vi "Read New Top Layer ID.vi"(8 "error in (no error)":errorcluster, 11 "Database Entry in":refnum<class "Database Entry.lvclass">) -> (0 "error out":errorcluster, 2 "Revised Sensor IDs":string[](array[string]), 3 "Database Entry out":refnum<class "Database Entry.lvclass">)   [LabVIEW 2021, in "Database Entry.lvclass"]
uses:
  Database Entry.lvclass
  Database Entry.lvclass/Database Entry.ctl
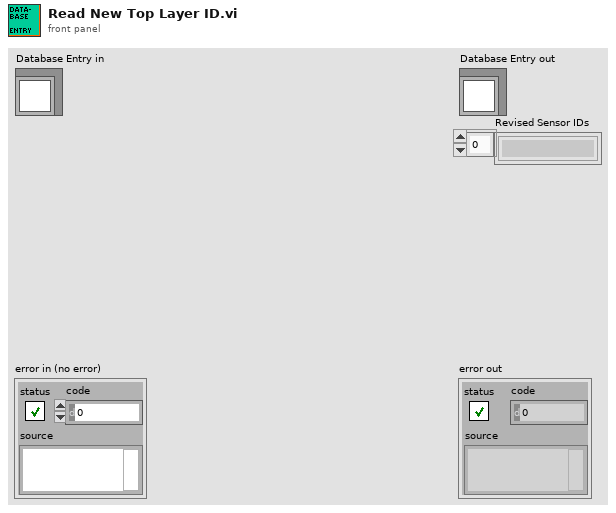
[diagram p1: front panel]
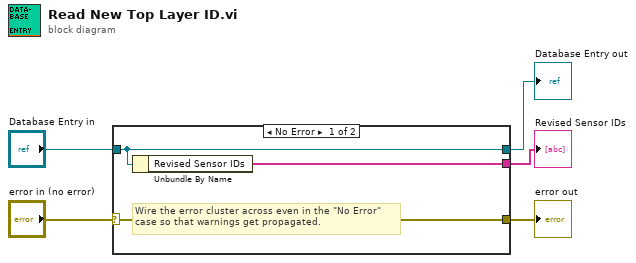
[diagram p0: block diagram]
diagram:
  n1 = case shown="No Error" "error in (no error)" {
    selector: "error in (no error)" -> [w8 w10]
    tunnel: [w8 w10] -> w4
    tunnel: [w7 w9] -> w2
    tunnel: "Database Entry in" -> [w7 w9]
    tunnel: [w6 _] -> w1
    frame No Error {
      # "Wire the error cluster across even in the \"No Error\"\ncase so that warnings get propagated."
      n2 = Unbundle By Name(w7) -> ("Revised Sensor IDs"=w6:string[])
    }
    frame Error {
    }
  }
  "error out" <- w4
  "Database Entry out" <- w2
  "Revised Sensor IDs" <- w1
